vi "SCT Initialize Dialog.vi"(6 "Time Triggered?":bool caption="时间触发？", 7 "Network Variables Only?":bool caption="只对网络变量？", 8 "error in (no error)":errorcluster caption="错误输入（无错误）", 11 "Variable Dialog Controls":T7 caption="变量对话控件") -> (0 "error out":errorcluster caption="错误输出", 1 "feature pack info":T2 caption="功能包信息", 2 "default types":T5 caption="默认类型", 3 "Variable Dialog Controls out":T7 caption="变量对话控件输出", 4 "broadcast event":T1 caption="广播事件", 5 "main loop broadcast listener":T1 caption="主循环广播侦听器")   [LabVIEW 2016]
uses:
  <resource>/dialog/variable/SCT Variable Dialog Controls.ctl
  <resource>/dialog/variable/SCT Default Types.ctl
  <vilib>/variable/Type Descriptor.ctl
  <resource>/dialog/variable/SCT Feature Pack Info.ctl
  <resource>/dialog/variable/SCT Message User Event.ctl
  <resource>/dialog/variable/SCT Message.ctl
  <resource>/dialog/variable/SCT Attributes.ctl
  <resource>/dialog/variable/SCT Attributes Event.ctl
  <resource>/dialog/variable/SCT Broadcast User Event.ctl
  <resource>/dialog/variable/SCT Broadcast.ctl
  <vilib>/variable/NI_Variable.lvlib
panel:
  in  "DataTypeLastElement (RTE)":string="来自LabVIEW自定义控件..." caption="数据类型最后一个元素(RTE)"
  in  "DataTypeLastElement":string="来自自定义控件..." caption="数据类型最后一个元素"
  # "用于本地化"
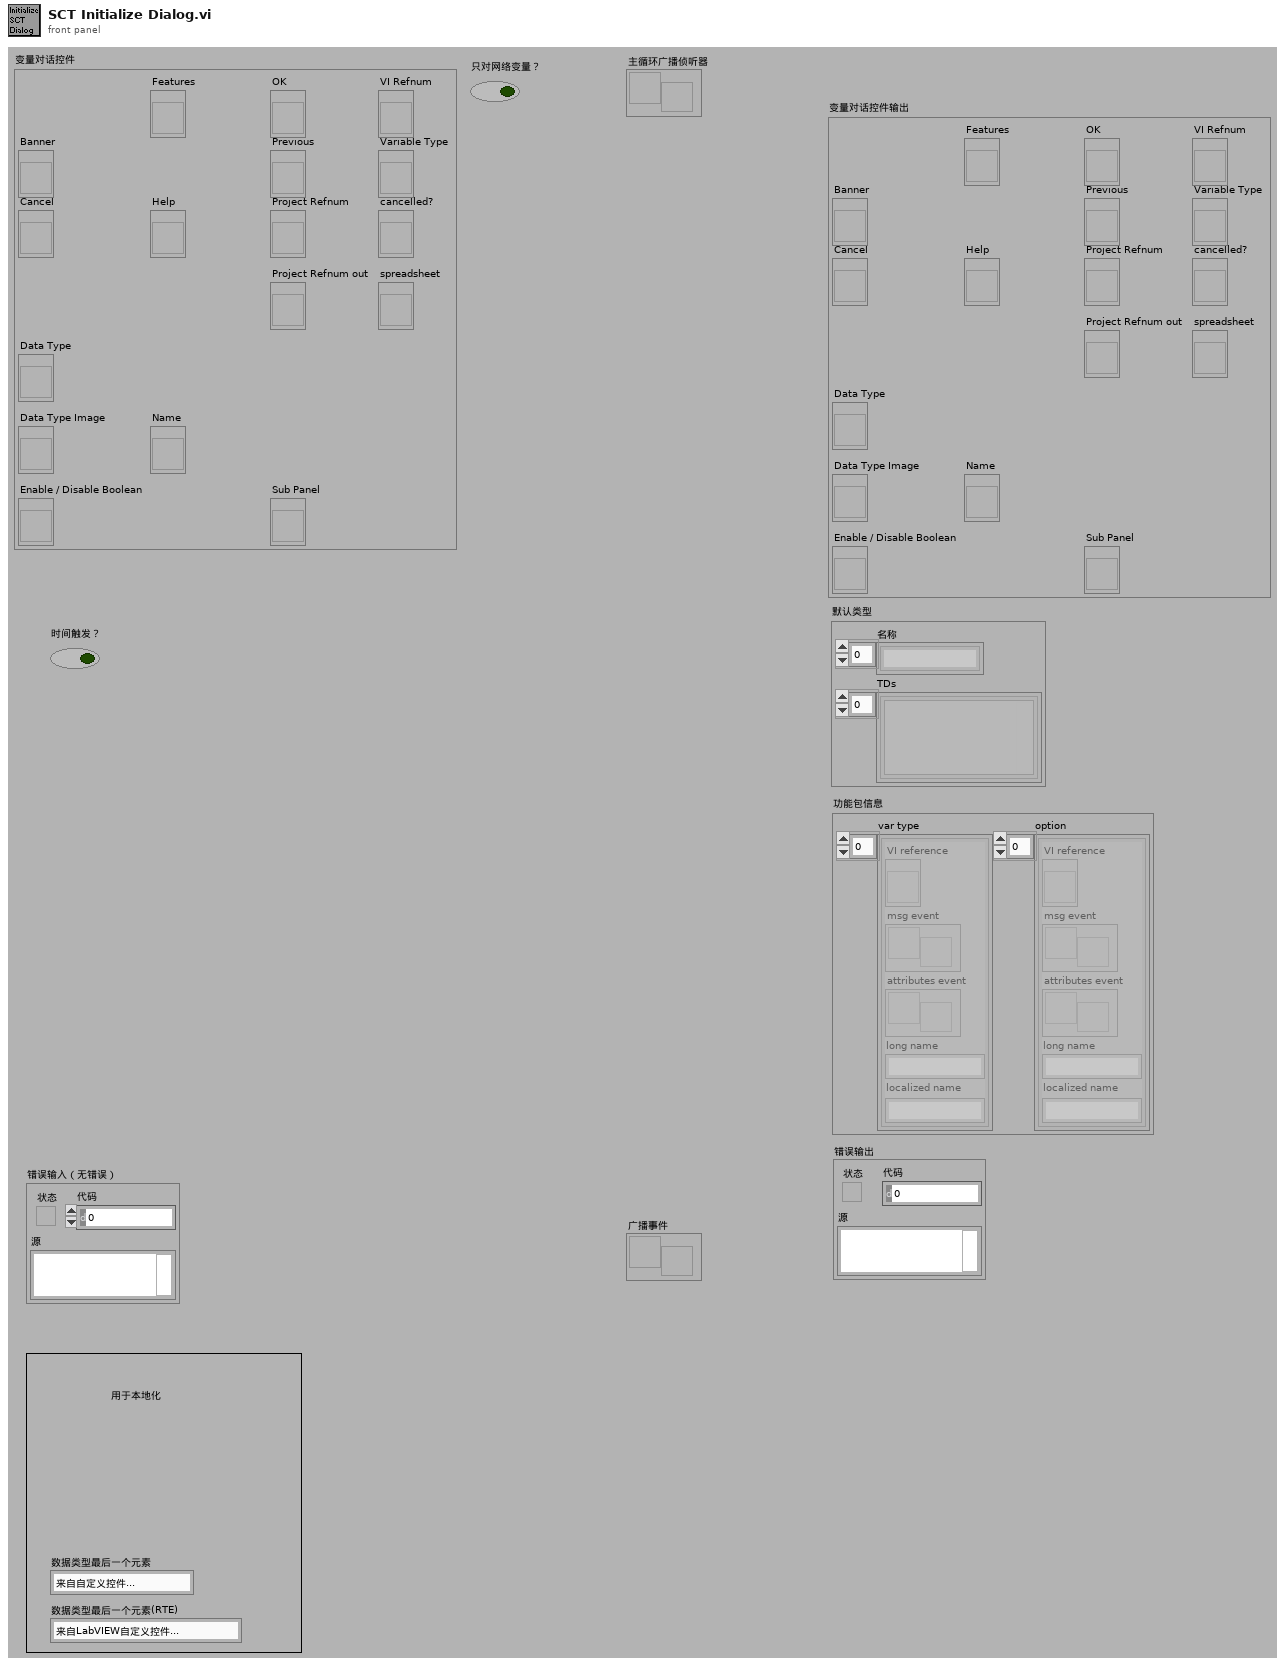
[diagram p1: front panel]
types:
  T1 = typedef "SCT Broadcast User Event.ctl" = refnum<user-event>
  T2 = typedef "SCT Feature Pack Info.ctl" = cluster{"var type":cluster{"VI reference":refnum<vi>, "msg event":T3, "attributes event":T4, "long name":string, "localized name":string}[], "option":cluster{"VI reference":refnum<vi>, "msg event":T3, "attributes event":T4, "long name":string, "localized name":string}[]}
  T3 = typedef "SCT Message User Event.ctl" = refnum<user-event>
  T4 = typedef "SCT Attributes Event.ctl" = refnum<user-event>
  T5 = typedef "SCT Default Types.ctl" = cluster{"names":string[], "TDs":T6[]}
  T6 = typedef "NI_Variable.lvlib/Type Descriptor.ctl" = cluster{"Variant":variant}
  T7 = typedef "SCT Variable Dialog Controls.ctl" = cluster{"Banner":refnum<vi>, "Cancel":refnum<vi>, "Data Type":refnum<vi>, "Data Type Image":refnum<vi>, "Enable / Disable Boolean":refnum<vi>, "Features":refnum<vi>, "Help":refnum<vi>, "Name":refnum<vi>, "OK":refnum<vi>, "Previous":refnum<vi>, "Project Refnum":refnum<vi>, "Project Refnum out":refnum<vi>, "Sub Panel":refnum<vi>, "VI Refnum":refnum<vi>, "Variable Type":refnum<vi>, "cancelled?":refnum<vi>, "spreadsheet":refnum<vi>}
  T8 = enum32{"invalid app kind", "Development System", "Run Time System", "Student Edition", "Embedded LabVIEW", "Evaluation", "Custom"}
  T9 = typedef "SCT Broadcast.ctl" = cluster{"name":string, "value":variant}
  T10 = cluster{"Enable / Disable Boolean":refnum<vi>, "Banner":refnum<vi>, "Sub Panel":refnum<vi>, refnum<vi>[]}
  T11 = cluster{"Name":refnum<vi>, "Variable Type":refnum<vi>, "Data Type":refnum<vi>, "Data Type Image":refnum<vi>, "Features":refnum<vi>, "OK":refnum<vi>, "Cancel":refnum<vi>}
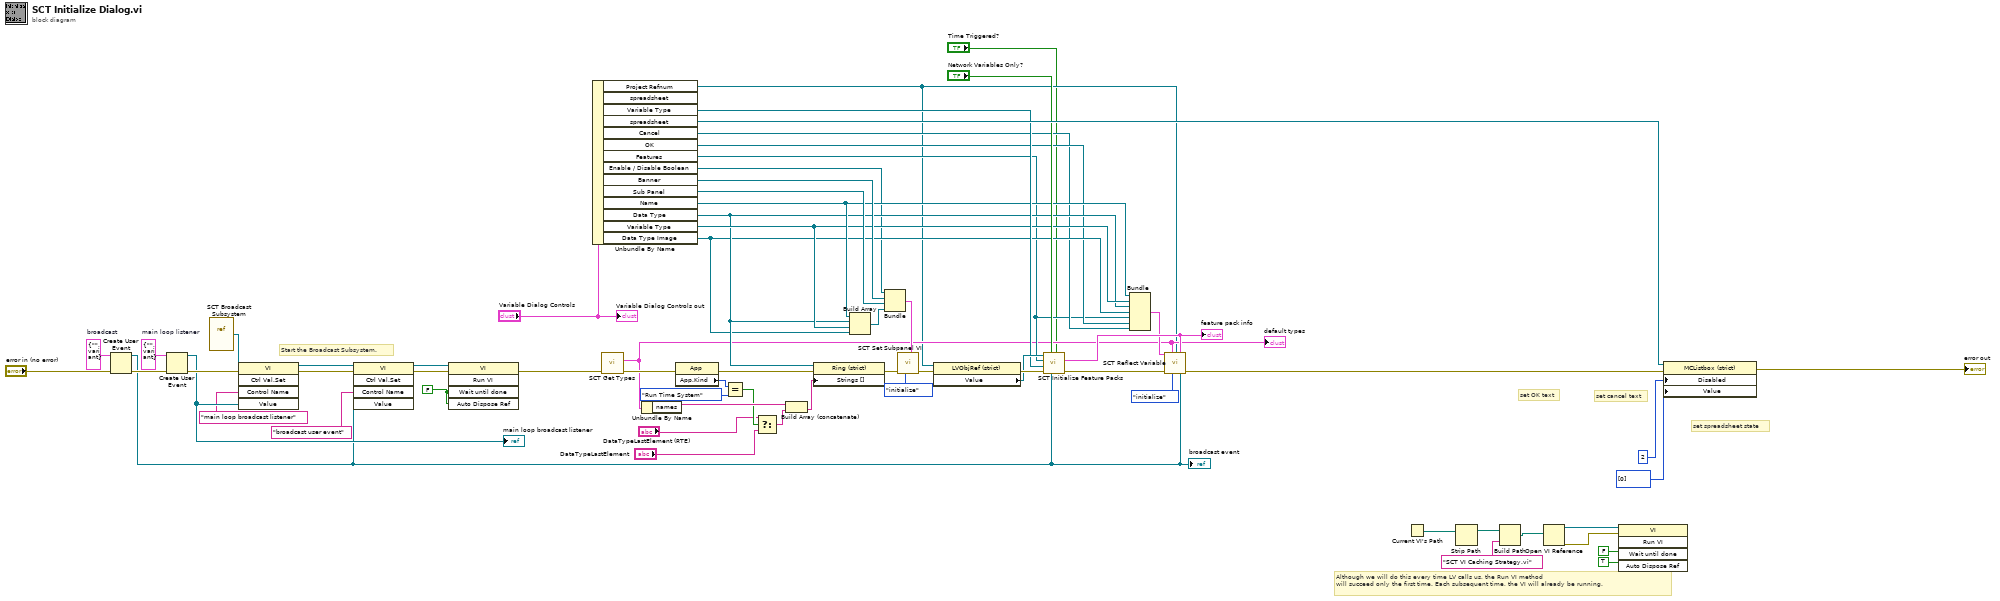
[diagram p0: block diagram]
diagram:
  w20 = FALSE ("Wait Until Done")
  w47 = T9 {"name"="", "value"=variant}  # main loop listener
  w48 = T9 {"name"="", "value"=variant}  # broadcast
  # "Start the Broadcast Subsystem."
  # "Although we will do this every time LV calls us, the Run VI method\nwill succeed only the first time. Each subsequent time, the VI will already be running."
  # "set spreadsheet state"
  # "set cancel text"
  # "set OK text"
  n1 = Create User Event(user event datatype=w48, error in="error in (no error)") -> (user event=w16:refnum<user-event>, error out=w46:errorcluster)
  "broadcast event" <- w16
  n2 = Create User Event(user event datatype=w47, error in=w46) -> (user event=w18:refnum<user-event>, error out=w21:errorcluster)
  "main loop broadcast listener" <- w18
  n3 = vi-ref <resource>:"SCT Broadcast Subsystem.vi"() -> (w19:refnum<vi>)
  n4 = invoke class="VI" method="Ctrl Val.Set"(reference=w19, error in=w21, "Control Name"="main loop broadcast listener", "Value"=w18) -> (reference out=w22:refnum<vi>, error out=w23:errorcluster)  [unwired: 1 in, 3 out]
  n5 = invoke class="VI" method="Ctrl Val.Set"(reference=w22, error in=w23, "Control Name"="broadcast user event", "Value"=w16) -> (reference out=w24:refnum<vi>, error out=w25:errorcluster)  [unwired: 1 in, 3 out]
  n6 = invoke class="VI" method="Run VI"(reference=w24, error in=w25, "Wait until done"=w20, "Auto Dispose Ref"=w20) -> (error out=w4:errorcluster)  [unwired: 1 in, 4 out]
  n7 = Unbundle By Name("Variable Dialog Controls") -> ("Project Refnum"=w2:refnum<vi>, "Variable Type"=w40:refnum<vi>, "spreadsheet"=w61:refnum<vi>, "Cancel"=w30:refnum<vi>, "OK"=w31:refnum<vi>, "Features"=w28:refnum<vi>, "Enable / Disable Boolean"=w32:refnum<vi>, "Banner"=w64:refnum<vi>, "Sub Panel"=w65:refnum<vi>, "Name"=w36:refnum<vi>, "Data Type"=w34:refnum<vi>, "Variable Type"=w35:refnum<vi>, "Data Type Image"=w33:refnum<vi>)  [unwired: 1 out]
  n8 = call <resource>:"SCT Get Types.vi"("error in"=w4) -> ("error out"=w50:errorcluster, "default types"=w14:T5)  [unwired: 8 in, 1 out]
  "default types" <- w14
  n9 = Unbundle By Name(w14) -> ("names"=w49:string[])
  n10 = property class="App"(error in=w50) -> (error out=w13:errorcluster, "App.Kind"=w12:T8)  [unwired: 1 in, 1 out]
  n11 = Equal?(x=w12, y=T8."Run Time System" ("Application:Kind")) -> (x = y?=w9:bool)
  n12 = Select(t="DataTypeLastElement (RTE)", s=w9, f="DataTypeLastElement") -> (s? t:f=w10:string)
  n13 = Build Array (concatenate)(w49, w10) -> (w26:string[])
  n14 = property on="Property Node" class="Ring (strict)"(reference=w34, error in=w13, "Strings []"=w26) -> (error out=w51:errorcluster)  [unwired: 1 out]
  n15 = Build Array(w36, w34, w35, w33) -> (w66:refnum<vi>[])
  n16 = Bundle("Enable / Disable Boolean"=w32, "Banner"=w64, "Sub Panel"=w65, w66) -> (w63:T10)  [unwired: 1 in]
  n17 = call <resource>:"SCT Set Subpanel VI.vi"("refnums"=w63, "operation"=enum16{"initialize", "set VI"}."initialize", "error in (no error)"=w51) -> ("error out"=w43:errorcluster)  [unwired: 8 in]
  n18 = property class="LVObjRef (strict)"(reference=w2, error in=w43) -> (error out=w42:errorcluster, "Value"=w41:refnum<vi>)  [unwired: 1 out]
  n19 = call <resource>:"SCT Initialize Feature Packs.vi"("Time-Triggered?"="Time Triggered?", "broadcast user event"=w16, "network variables only"="Network Variables Only?", "error in (no error)"=w42, "variable type ring"=w40, "feature listbox"=w28, "Project Refnum"=w41) -> ("error out"=w39:errorcluster, "feature pack info"=w38:T2)  [unwired: 3 in]
  "feature pack info" <- w38
  n20 = Bundle("Name"=w36, "Variable Type"=w35, "Data Type"=w34, "Data Type Image"=w33, "Features"=w28, "OK"=w31, "Cancel"=w30) -> (w29:T11)  [unwired: 1 in]
  n21 = call <resource>:"SCT Reflect Variable.vi"("refnums"=w29, "default types"=w14, "Project Refnum"=w2, "feature pack info"=w38, "error in (no error)"=w39, "operation"=enum16{"initialize", "reflect"}."initialize", "broadcast user event"=w16) -> ("error out"=w6:errorcluster)  [unwired: 5 in, 3 out]
  n22 = Current VI's Path() -> (path=w52:path)
  n23 = Strip Path(path=w52) -> (stripped path=w54:path)  [unwired: 1 out]
  n24 = Build Path(base path=w54, name or relative path="SCT VI Caching Strategy.vi") -> (appended path=w55:path)
  n25 = Open VI Reference(vi path=w55) -> (vi reference=w56:refnum<vi>, error out=w59:errorcluster)  [unwired: 5 in]
  n26 = invoke class="VI" method="Run VI"(reference=w56, error in=w59, "Wait until done"=FALSE ("Wait Until Done"), "Auto Dispose Ref"=TRUE ("Auto Dispose Reference")) -> ()  [unwired: 1 in, 5 out]
  n27 = property on="Property Node" class="MCListbox (strict)"(reference=w61, error in=w6, "Disabled"=u8 2, "Value"=i32[] [0] ("spreadsheet")) -> (error out=→"error out":errorcluster)  [unwired: 1 out]
  "Variable Dialog Controls out" <- "Variable Dialog Controls"
